vi "parseXMLstring.vi"(8 "error in (no error)":errorcluster, 10 "Node Value":string, 11 "Experiment.lvclass (in)":refnum<class "Experiment.lvclass">) -> (0 "error out":errorcluster, 3 "Experiment.lvclass":refnum<class "Experiment.lvclass">)   [LabVIEW 2014, in "Experiment.lvclass"]
uses:
  Experiment.lvclass
  Experiment.lvclass/Experiment.ctl
  Globals.vi
  <vilib>/xml/Close Reference(Node).vi
  DDS/DDS.lvclass
  <vilib>/xml/NI_XML.lvlib
  <resource>/objmgr/DOMUserDefRef.rc
  TCP_IP/TCP_IP.lvclass
panel:
  out "Parse Errors":string
  out "Display of element names":string[](array[string])
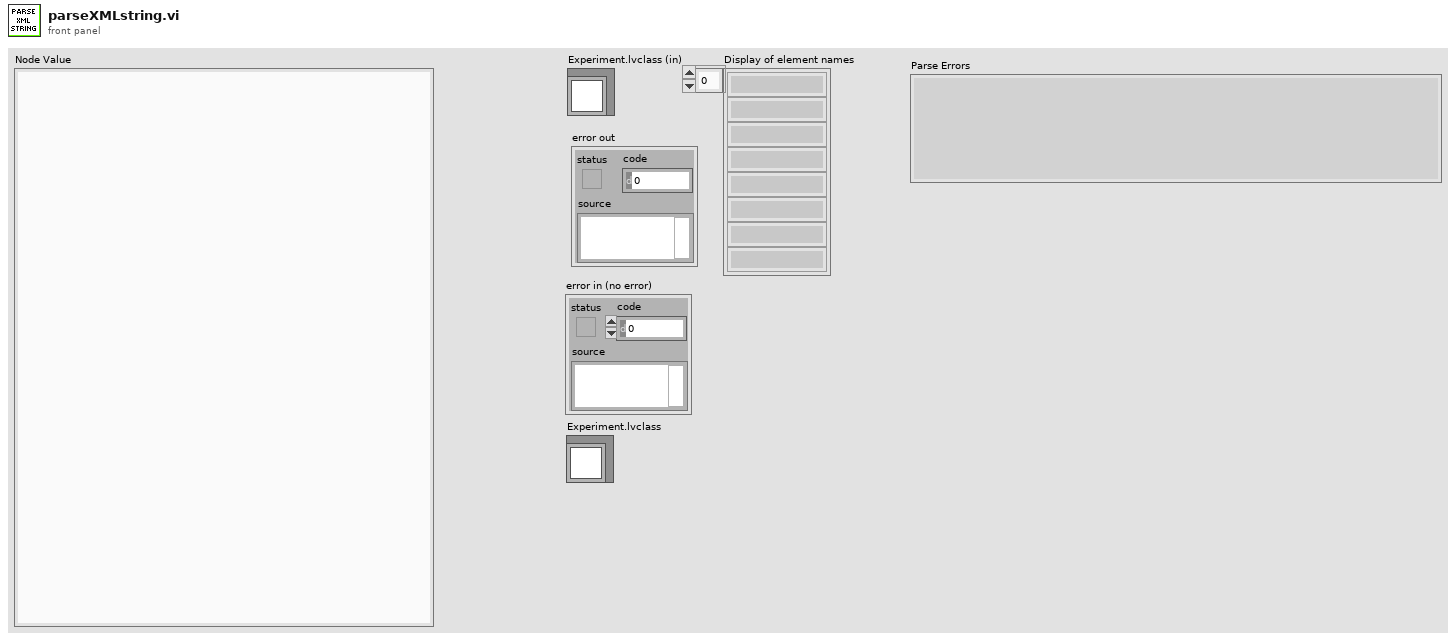
[diagram p1: front panel]
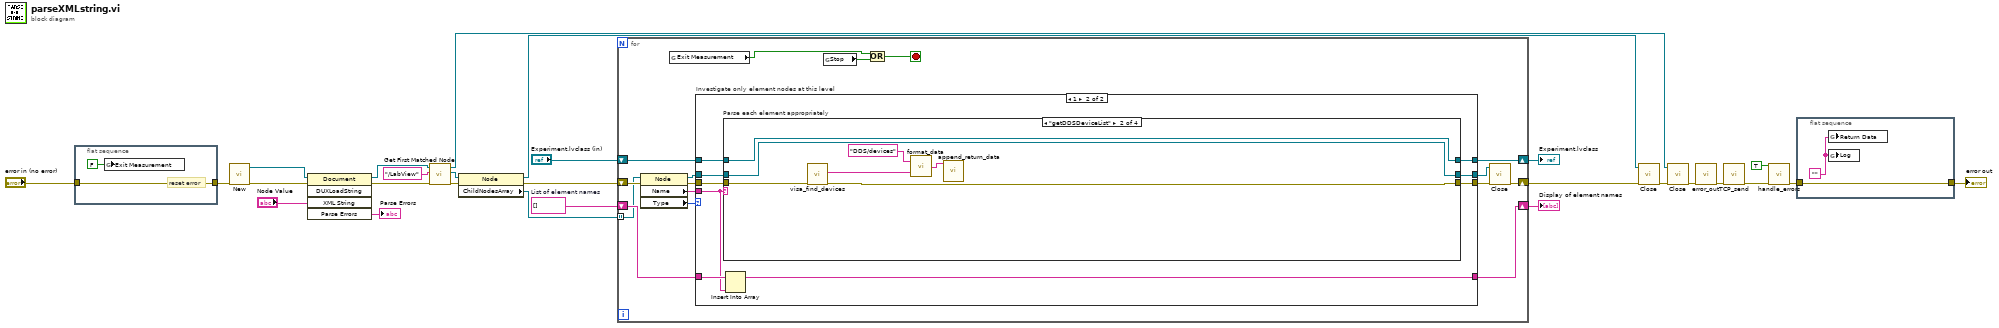
[diagram p0: block diagram]
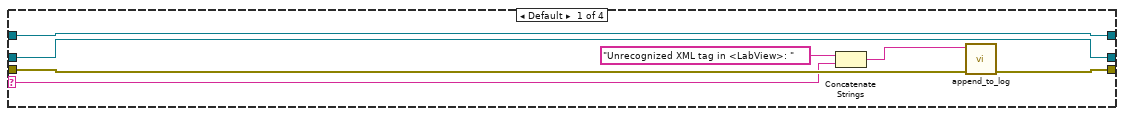
[diagram p3: hidden frame]
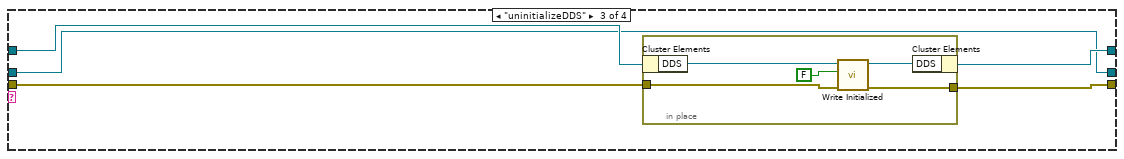
[diagram p4: hidden frame]
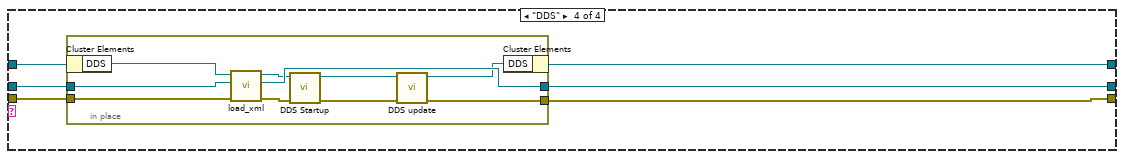
[diagram p5: hidden frame]
diagram:
  w19 = string[] []  # List of element names
  n1 = flat-sequence {
    tunnel: "error in (no error)" -> [w29]
    tunnel: [w29] -> w7
    frame #0 {
      # "reset error"
      n2 = global write "Globals.vi" "Exit Measurement"(FALSE ("Exit Measurement")) -> ()
    }
  }
  n3 = call <vilib>:"New.vi"("error in (no error)"=w7) -> ("error out"=w12:errorcluster, "DOM document out"=w20:refnum<k20>)  [unwired: 7 in]
  n4 = invoke class="Document" method="DUXLoadString"(reference=w20, error in=w12, "XML String"="Node Value") -> (reference out=w23:refnum<k20>, error out=w11:errorcluster, "Parse Errors"=→"Parse Errors":string)  [unwired: 2 in, 2 out]
  n5 = call <vilib>:"Get First Matched Node.vi"("error in (no error)"=w11, "XPath expression"="/LabView", "node in"=w23) -> ("error out"=w17:errorcluster, "node result"=w13:refnum<k20>, "node out"=w18:refnum<k20>)  [unwired: 6 in]
  n6 = property class="Node"(reference=w13, error in=w17) -> (reference out=w21:refnum<k20>, error out=w15:errorcluster, "ChildNodesArray"=w27:refnum<k20>[])
  n7 = for {
    tunnel: w27 -> [w39] mode=indexing
    shift-right: [w42] -> w26
    shift-left: w19 -> [w43]
    shift-right: [w41] -> w16
    shift-left: w15 -> [w40]
    shift-right: [w33] -> w9
    shift-left: "Experiment.lvclass (in)" -> [w34]
    stop <- w30 stop-if-true
    n8 = property class="Node"(reference=w39, error in=w40) -> (reference out=w36:refnum<k20>, error out=w38:errorcluster, "Name"=w44:string, "Type"=w45:i32)
    n9 = global read "Globals.vi" "Exit Measurement"() -> (w32:bool)
    n10 = case "Investigate only element nodes at this level" shown="1" w45 {
      tunnel: w44 -> [_ w56]
      tunnel: w43 -> [w49 w58]
      tunnel: [w49 w57] -> w42
      tunnel: w36 -> [w47 w55]
      tunnel: w38 -> [w48 w54]
      tunnel: [w48 w53] -> w37
      tunnel: [w47 w52] -> w35
      tunnel: w34 -> [w46 w51]
      tunnel: [w46 w50] -> w33
      frame Default {
      }
      frame 1 {
        n11 = case "Parse each element appropriately" shown="\"getDDSDeviceList\"" w56 {
          selector: w56 -> [w62 _ _ _]
          tunnel: w55 -> [w60 w69 w73 w84]
          tunnel: w54 -> [w65 w68 w75 w85]
          tunnel: [w64 w67 w74 w86] -> w53
          tunnel: [w60 w69 w73 w83] -> w52
          tunnel: w51 -> [w59 w70 w77 w88]
          tunnel: [w59 w70 w76 w87] -> w50
          frame Default {
            n12 = Concatenate Strings("Unrecognized XML tag in <LabView>: " ("string"), w62) -> (w61:string)
            n13 = call "append_to_log.vi"("error in"=w65, "string"=w61) -> ("error out"=w64:errorcluster)  [unwired: 9 in]
          }
          frame "getDDSDeviceList" {
            n14 = call "visa_find_devices.vi"("error in (no error)"=w68) -> ("error out"=w67:errorcluster, "devices found string"=w66:string)  [unwired: 8 in, 1 out]
            n15 = call "format_data.vi"("data"=w66, "name"="DDS/devices") -> ("concatenated string"=w71:string)
            n16 = call "append_return_data.vi"("Return Data"=w71) -> ()  [unwired: 11 in]
          }
          frame "uninitializeDDS" {
            n17 = in-place {
              in-place-border: w75 -> [w79]
              in-place-border: [w78] -> w74
              n18 = in-place-cluster #1(w77) -> ("DDS"=w82:refnum<class "DDS.lvclass">)
              n19 = call-dynamic "Write Initialized.vi"("error in (no error)"=w79, "Initialized"=FALSE, "DDS in"=w82) -> ("error out"=w78:errorcluster, "DDS out"=w81:refnum<class "DDS.lvclass">)  [unwired: 7 in]
              n20 = in-place-cluster #1("DDS"=w81) -> (w76:refnum<class "Experiment.lvclass">)
            }
          }
          frame "DDS" {
            n21 = in-place {
              in-place-border: [w93] -> w86
              in-place-border: w85 -> [w96]
              in-place-border: w84 -> [w97]
              in-place-border: [w95] -> w83
              n22 = in-place-cluster #2(w88) -> ("DDS"=w98:refnum<class "DDS.lvclass">)
              n23 = call "load_xml.vi"("error in"=w96, "child node in"=w97, "DDS.lvclass (in)"=w98) -> ("error out"=w91:errorcluster, "child node out"=w95:refnum<k20>, "DDS.lvclass"=w92:refnum<class "DDS.lvclass">)  [unwired: 6 in]
              n24 = call "DDS Startup.vi"("error in (no error)"=w91, "DDS.lvclass (in)"=w92) -> ("error out"=w90:errorcluster, "DDS.lvclass"=w89:refnum<class "DDS.lvclass">)  [unwired: 8 in]
              n25 = call "DDS update.vi"("error in (no error)"=w90, "DDS.lvclass (in)"=w89) -> ("error out"=w93:errorcluster, "DDS.lvclass"=w94:refnum<class "DDS.lvclass">)  [unwired: 8 in]
              n26 = in-place-cluster #2("DDS"=w94) -> (w87:refnum<class "Experiment.lvclass">)
            }
          }
        }
        n27 = Insert Into Array(array=w58, new element=w56) -> (w57:string[])  [unwired: 1 in]
      }
    }
    n28 = global read "Globals.vi" "Stop"() -> (w31:bool)
    n29 = Or(x=w32, y=w31) -> (x .or. y?=w30:bool)
    n30 = call-poly <vilib>:"Close.vi"("error in (no error)"=w37, "node"=w35) -> ("error out"=w41:errorcluster)  [unwired: 7 in]
  }
  "Display of element names" <- w26
  "Experiment.lvclass" <- w9
  n31 = call-poly <vilib>:"Close.vi"("error in (no error)"=w16, "node"=w21) -> ("error out"=w14:errorcluster)  [unwired: 7 in]
  n32 = call-poly <vilib>:"Close.vi"("error in (no error)"=w14, "node"=w18) -> ("error out"=w5:errorcluster)  [unwired: 7 in]
  n33 = call "error_out.vi"("error in (no error)"=w5) -> ("error out"=w6:errorcluster)  [unwired: 10 in]
  n34 = call "TCP_send.vi"("error in (no error)"=w6) -> ("error out"=w4:errorcluster)  [unwired: 10 in]
  n35 = call "handle_errors.vi"("Exit Operation"=TRUE ("Exit Measurement"), "error in (no error)"=w4) -> ("error out"=w1:errorcluster)  [unwired: 13 in]
  n36 = flat-sequence {
    tunnel: [w100] -> w2
    tunnel: w1 -> [w100]
    frame #0 {
      w99 = ""
      n37 = global write "Globals.vi" "Return Data"(w99) -> ()
      n38 = global write "Globals.vi" "Log"(w99) -> ()
    }
  }
  "error out" <- w2
